vi "Clear Errors.vi"(4 "error in (no error)":errorcluster) -> (0 "error out":errorcluster)   [LabVIEW 2010]
doc: "Resets the error <B>status</B> to no error, <B>code</B> to 0, and <B>source</B> to an empty string. Use this VI when you want to ignore an error."
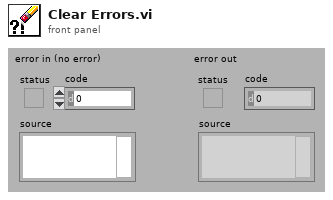
[diagram p1: front panel]
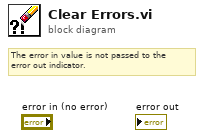
[diagram p0: block diagram]
diagram:
  # "The error in value is not passed to the\nerror out indicator."
